vi "Deccel.vi"(6 "MotrSpdInfo":T1) -> (3 "SpdMult":dbl)   [LabVIEW 2017]
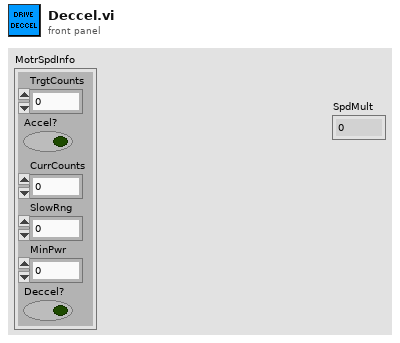
[diagram p1: front panel]
types:
  T1 = cluster{"TrgtCounts":i32, "Accel?":bool, "CurrCounts":dbl, "SlowRng":dbl, "MinPwr":dbl, "Deccel?":bool}
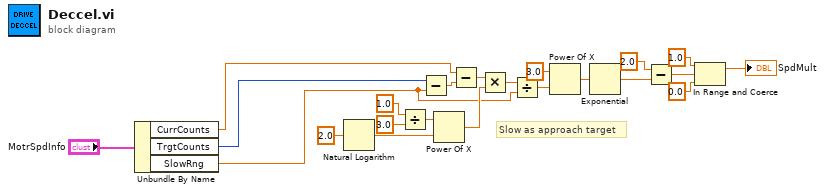
[diagram p0: block diagram]
diagram:
  # "Slow as approach target"
  n1 = Unbundle By Name("MotrSpdInfo") -> ("CurrCounts"=w3:dbl, "TrgtCounts"=w4:i32, "SlowRng"=w5:dbl)
  n2 = Natural Logarithm(1:2.0 ("x")) -> (0:w11:dbl)
  n3 = Divide(x=1.0, y=3.0 ("x")) -> (x/y=w12:dbl)
  n4 = Subtract(x=w4, y=w5) -> (x-y=w8:dbl)
  n5 = Power Of X(1:w11, 2:w12) -> (0:w15:dbl)
  n6 = Subtract(x=w3, y=w8) -> (x-y=w9:dbl)
  n7 = Multiply(x=w9, y=w15) -> (x*y=w16:dbl)
  n8 = Divide(x=w16, y=w5) -> (x/y=w17:dbl)
  n9 = Power Of X(1:w17, 2:3.0 ("x")) -> (0:w19:dbl)
  n10 = Exponential(1:w19) -> (0:w20:dbl)
  n11 = Subtract(x=2.0, y=w20) -> (x-y=w7:dbl)
  n12 = In Range and Coerce(upper limit=1.0 ("f"), x=w7, lower limit=0.0 ("f")) -> (coerced(x)=→"SpdMult":dbl)  [unwired: 1 out]
